vi "Read SubComponent Parameter - Scaled.vi"(8 "error in (no error)":errorcluster, 10 "Parameter":string, 11 "1553 SubComponent in":refnum<class "1553 SubComponent.lvclass">) -> (0 "error out":errorcluster, 2 "Scaled Data":dbl)   [LabVIEW 2020, in "BCI-1553 API.lvlib" / "1553 SubComponent.lvclass"]
doc: "Reads a scaled value for a single parameter, as opposed to all the parameters at once."
uses:
  1553 SubComponent.lvclass
  Frames & Messages/TypeDefs/Parameter Table Data.ctl
  Frames & Messages/TypeDefs/Scaling Information.ctl
  1553 SubComponent.lvclass/1553 SubComponent.ctl
  Dependencies/Registry/Registry.lvclass/Registry.ctl
  Dependencies/Registry/Registry.lvclass
  BCI-1553 API.lvlib
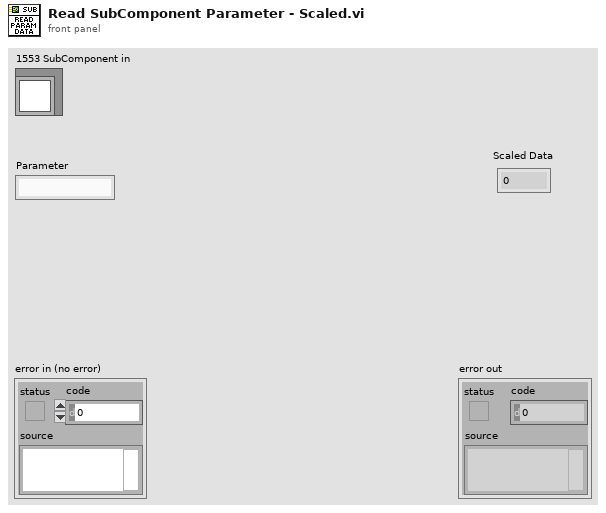
[diagram p1: front panel]
types:
  T1 = typedef "BCI-1553 API.lvlib/Parameter Table Data.ctl" = cluster{"Parameter Name":string, "Base Word":u16, "Address":u16, "Value":u64, "Mask":u16[], "Scaling Info":T2}
  T2 = typedef "BCI-1553 API.lvlib/Scaling Information.ctl" = cluster{"Bit Offset":i32, "Bit Count":i32, "LSB Resolution":dbl, "2's Complement":bool, "Big Endian":bool, "Sign Bit":bool}
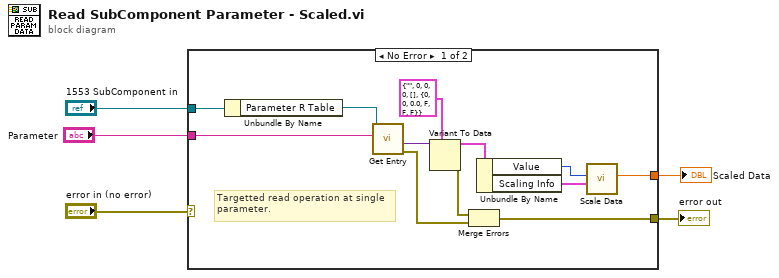
[diagram p0: block diagram]
diagram:
  n1 = case shown="No Error" "error in (no error)" {
    selector: "error in (no error)" -> [_ w18]
    tunnel: [w6 w18] -> w4
    tunnel: "1553 SubComponent in" -> [w13 _]
    tunnel: "Parameter" -> [w12 _]
    tunnel: [w9 _] -> w1
    frame No Error {
      # "Targetted read operation at single\nparameter."
      n2 = Unbundle By Name(w13) -> ("Parameter R Table"=w17:refnum<class "Registry.lvclass">)
      n3 = call "Get Entry.vi"("Key"=w12, "Registry in"=w17) -> ("error out"=w7:errorcluster, "Value"=w15:variant)  [unwired: 6 in, 2 out]
      n4 = Variant To Data(type=T1 {"Parameter Name"="", "Base Word"=0, "Address"=0, "Value"=0, "Mask"=[], "Scaling Info"={"Bit Offset"=0, "Bit Count"=0, "LSB Resolution"=0.0, "2's Complement"=FALSE, "Big Endian"=FALSE, "Sign Bit"=FALSE}} ("Parameter Table Data"), Variant=w15) -> (data=w16:T1, error out=w8:errorcluster)  [unwired: 1 in]
      n5 = Merge Errors(w8, w7) -> (w6:errorcluster)
      n6 = Unbundle By Name(w16) -> ("Value"=w10:u64, "Scaling Info"=w11:T2)
      n7 = call "Scale Data.vi"("Scaling Info"=w11, "Raw Value"=w10) -> ("Scaled Value"=w9:dbl)  [unwired: 8 in, 1 out]
    }
    frame Error {
    }
  }
  "error out" <- w4
  "Scaled Data" <- w1
